vi "solar Create (Target).vi"(8 "error in (no error)":errorcluster, 10 "Target Name":string, 11 "Default LVClass":refnum<class "solar.lvclass">) -> (0 "error out":errorcluster, 3 "solar":refnum<class "solar.lvclass">)   [LabVIEW 2018, in "solar.lvclass"]
doc: "This loads the target's queue reference from the global SOLAR reference. All SOLAR targets are stored in a single element queue. \nNote: This VI does not create the Target queue if it does not exist."
uses:
  solar.lvclass
  solar_ctl SOLAR Global.ctl
  solar_ctl Target Global.ctl
  voyager/solar_voy_ctl Voyager Refnum.ctl
  qtimer/solar_qtimer_ctl Refnum.ctl
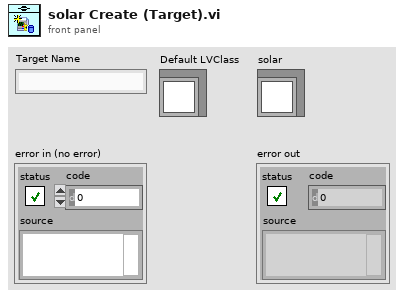
[diagram p1: front panel]
types:
  T1 = typedef "solar_ctl SOLAR Global.ctl" = cluster{"Targets":T2[], "AppDir":path, "solar.ini":path, "ConfigsDir":path, "CosmosDir":path, "LogsDir":path, "ExePath":path, "ExeVersion":string, "PartNum":string, "AppSetup":string, "Title":string, "Main.ini":path, "Temp.ini":path, "vSOLAR":string, "Splash.png":string, "SplashWait":i32, "SOLARUE":refnum<user-event>, "VoyagerRefnum":T3, "QTimerRefnum":T4}
  T2 = typedef "solar_ctl Target Global.ctl" = cluster{"Target":string, "Q":refnum<queue>, "UE":refnum<user-event>, "VI":refnum<vi>, "Menu":refnum<k9>, "Data":refnum<data-value>, "Attributes":variant}
  T3 = typedef "solar_voy_ctl Voyager Refnum.ctl" = refnum<k1>
  T4 = typedef "solar_qtimer_ctl Refnum.ctl" = refnum<k1>
  T5 = typedef "solar_ctl SOLAR Refnum.ctl" = refnum<k1>
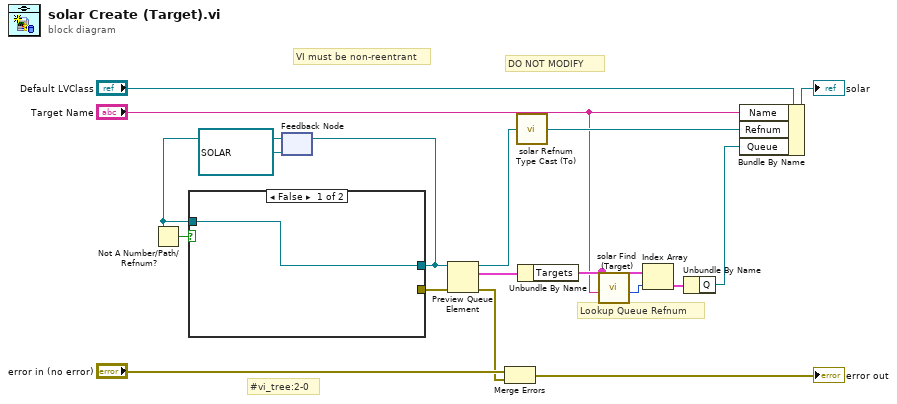
[diagram p0: block diagram]
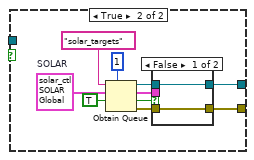
[diagram p2: hidden frame]
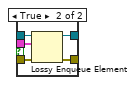
[diagram p3: hidden frame]
diagram:
  # "VI must be non-reentrant"
  # "#vi_tree:2-0"
  # "DO NOT MODIFY"
  # "Lookup Queue Refnum"
  n1 = feedback #1(refnum<queue> refnum ("queue out")) -> (w3:refnum<queue>)
  n2 = Not A Number/Path/Refnum?(number/path/refnum=w3) -> (NaN/Path/Refnum?=w2:bool)
  n3 = case shown="False" w2 {
    tunnel: [w19 w22] -> w1
    tunnel: [_ w20] -> w7
    tunnel: w3 -> [w19 _]
    frame False {
    }
    frame True {
      w23 = T1 {"Targets"=[], "AppDir"=path "", "solar.ini"=path "", "ConfigsDir"=path "", "CosmosDir"=path "", "LogsDir"=path "", "ExePath"=path "", "ExeVersion"="", "PartNum"="", "AppSetup"="", "Title"="", "Main.ini"=path "", "Temp.ini"=path "", "vSOLAR"="", "Splash.png"="", "SplashWait"=0, "SOLARUE"=refnum, "VoyagerRefnum"=refnum, "QTimerRefnum"=refnum}  # SOLAR
      n4 = Obtain Queue(max queue size (-1, unlimited)=1, name (unnamed)="solar_targets" ("string"), element data type=w23, create if not found? (T)=TRUE ("Create if not found? (T)")) -> (queue out=w25:refnum<queue>, created new?=w24:bool, error out=w21:errorcluster)  [unwired: 1 in]
      n5 = case shown="False" w24 {
        tunnel: w25 -> [w30 w35]
        tunnel: w23 -> [_ w34]
        tunnel: [w30 w33] -> w22
        tunnel: w21 -> [w29 w32]
        tunnel: [w29 w31] -> w20
        frame False {
        }
        frame True {
          n6 = Lossy Enqueue Element(queue=w35, element=w34, error in (no error)=w32) -> (queue out=w33:refnum<queue>, error out=w31:errorcluster)  [unwired: 2 out]
        }
      }
    }
  }
  n7 = feedback-in #1(w1) -> ()
  n8 = Preview Queue Element(queue=w1, error in (no error)=w7) -> (queue out=w13:refnum<queue>, element=w12:T1, error out=w6:errorcluster)  [unwired: 1 in, 1 out]
  n9 = Merge Errors("error in (no error)", w6) -> (→"error out":errorcluster)
  n10 = call "solar Refnum Type Cast (To).vi"("SOLAR"=w13) -> ("Refnum"=w17:T5)
  n11 = Unbundle By Name(w12) -> ("Targets"=w11:T2[])
  n12 = call "solar Find (Target).vi"("Target"="Target Name", "Targets"=w11) -> ("Target Index"=w10:i32)  [unwired: 8 in, 1 out]
  n13 = Index Array(array=w11, index=w10) -> (element=w9:T2)
  n14 = Unbundle By Name(w9) -> ("Q"=w8:refnum<queue>)
  n15 = Bundle By Name(cluster="Default LVClass", "Name"="Target Name", "Refnum"=w17, "Queue"=w8) -> (→"solar":refnum<class "solar.lvclass">)
